vi "FCE_TS_Action_CalculatedValues.vi"(8 "err in":errorcluster) -> (0 "err out":errorcluster)   [LabVIEW 2017]
uses:
  FCE_TS_General_Libs/Kirschenhofer_Libs/KH Turck EthernetIP 17.12/KH TURCK TypeDefs FGlob.ctl
  FCE_TS_FGlob_V001.llb/FCE_TS_FGlob_TDefEnum_Stream Write Items.ctl
  FCE_TS_Alarm_V001.llb/FCE_TS_Alarm_Globals.vi
  FCE_TS_FGlob_V001.llb/FCE_TS_FGlob_TDefEnumcDAQAIItems.ctl
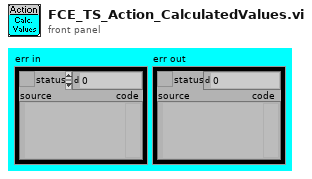
[diagram p1: front panel]
types:
  T1 = typedef "FCE_TS_FGlob_TDefEnum_Stream Write Items.ctl" = enum16{"Global State FCE_TS [-]", "Watchdog FCET FCE1 [-]", "Fp_CONT_FCET_AI [barg]", "Fp_HPRU_FCET_AI [barg]", "FT_CONT_FCET_AI [°C]", "Alarm Status FCET [-]"}
  T2 = typedef "KH TURCK TypeDefs FGlob.ctl" = enum16{"Put one", "Put all", "Recall one", "Recall all"}
  T3 = typedef "WL_Alarm_TypeDefClusterStatus.ctl" = cluster{"NOTAUS":bool, "ABSCHALTEN":bool, "MELDUNG":bool}
  T4 = typedef "FCE_TS_FGlob_TDefEnumcDAQAIItems.ctl" = enum16{"Fp_HPRU_TS1", "Fp_HPRU_TS2", "Fp_So_TS", "AT_EXH_TS", "EU_DCDCi_TS", "EI_DCDC24V_TS", "EI_DIV25A_TS", "EI_DCDC12V_TS", "EI_ETC_TS", "EI_DIV40A_TS", "EI_DCDCi_TS", "EI_DCDCo_TS", "EI_BAT_TS", "EI_LOAD_TS", "Reserve_AI_4_2", "Reserve_AI_4_3", "AT_Si_TS", "AT_So_TS", "CT_Si_TS", "CT_So_TS", "Ck_CP1i_TS", "Cp_CP1i_TS", "Cp_CP1o_TS", "Cp_CP2o_TS"}
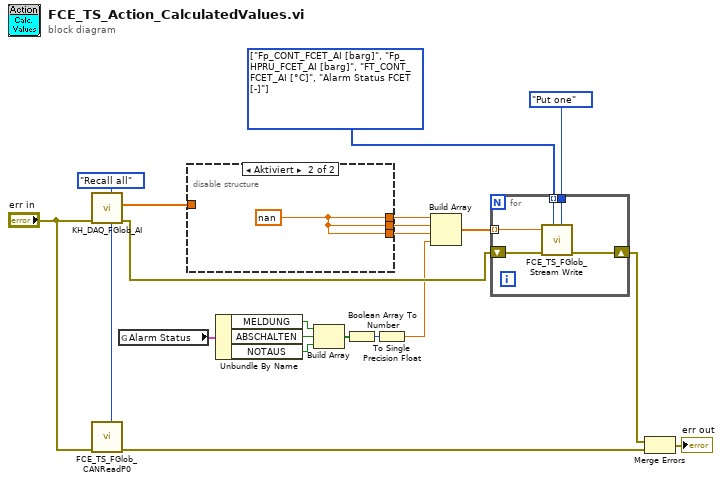
[diagram p0: block diagram]
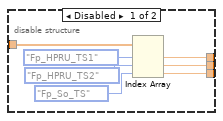
[diagram p2: hidden frame]
diagram:
  w12 = T1[] [enum."Fp_CONT_FCET_AI [barg]", enum."Fp_HPRU_FCET_AI [barg]", enum."FT_CONT_FCET_AI [°C]", enum."Alarm Status FCET [-]"] items=["Global State FCE_TS [-]", "Watchdog FCET FCE1 [-]", "Fp_CONT_FCET_AI [barg]", "Fp_HPRU_FCET_AI [barg]", "FT_CONT_FCET_AI [°C]", "Alarm Status FCET [-]"] ("Array")
  w20 = KH_TURCK_TypeDefs_FGlob."Recall all" ("Function (Recall One)")
  n1 = call "KH_DAQ_FGlob_AI.vi"("Function (Recall One)"=w20, "err in"="err in") -> ("err out"=w11:errorcluster, "AI Values OUT"=w17:sgl[])  [unwired: 6 in, 2 out]
  n2 = call "FCE_TS_FGlob_CANReadP0.vi"("Function (Recall One)"=w20, "err in"="err in") -> ("err out"=w9:errorcluster)  [unwired: 7 in, 2 out]
  n3 = global read "FCE_TS_Alarm_Globals.vi" "Alarm Status"() -> (w7:T3)
  n4 = disable-structure shown="Aktiviert" {
    disable-tunnel: w17 -> [w27 _]
    disable-tunnel: [w23 w28] -> w16
    disable-tunnel: [w22 w28] -> w15
    disable-tunnel: [w21 w28] -> w14
    frame Disabled {
      n5 = Index Array(array=w27, index #1=FCE_TS_FGlob_TDefEnumcDAQAIItems."Fp_HPRU_TS1" ("PXI_AI_Item"), index #2=FCE_TS_FGlob_TDefEnumcDAQAIItems."Fp_HPRU_TS2" ("PXI_AI_Item"), index #3=FCE_TS_FGlob_TDefEnumcDAQAIItems."Fp_So_TS" ("PXI_AI_Item")) -> (element #1=w23:sgl, element #2=w22:sgl, element #3=w21:sgl)
    }
    frame Enabled {
      w28 = sgl nan ("values")
    }
  }
  n6 = Unbundle By Name(w7) -> ("MELDUNG"=w6:bool, "ABSCHALTEN"=w5:bool, "NOTAUS"=w4:bool)
  n7 = Build Array(w6, w5, w4) -> (w3:bool[])
  n8 = Boolean Array To Number(Boolean array=w3) -> (number=w2:u32)
  n9 = To Single Precision Float(number=w2) -> (single precision float=w1:sgl)
  n10 = Build Array(w16, w15, w14, w1) -> (w13:sgl[])
  n11 = for {
    tunnel: KH_TURCK_TypeDefs_FGlob."Put one" ("Function (Recall One)") -> [w33]
    tunnel: w13 -> [w32] mode=indexing
    tunnel: w12 -> [w31] mode=indexing
    shift-right: [w29] -> w10
    shift-left: w11 -> [w30]
    n12 = call "FCE_TS_FGlob_Stream Write.vi"("Function (Recall One)"=w33, "Stream Write Items"=w31, "err in"=w30, "AI Value IN"=w32) -> ("err out"=w29:errorcluster)  [unwired: 5 in, 2 out]
  }
  n13 = Merge Errors(w10, w9) -> (→"err out":errorcluster)
